vi "Append Waveform Data.vi"(8 "Count":i32, 10 "Data In":waveform(dbl), 11 "Data":waveform(dbl)) -> (3 "Data Out":waveform(dbl))   [LabVIEW 2018]
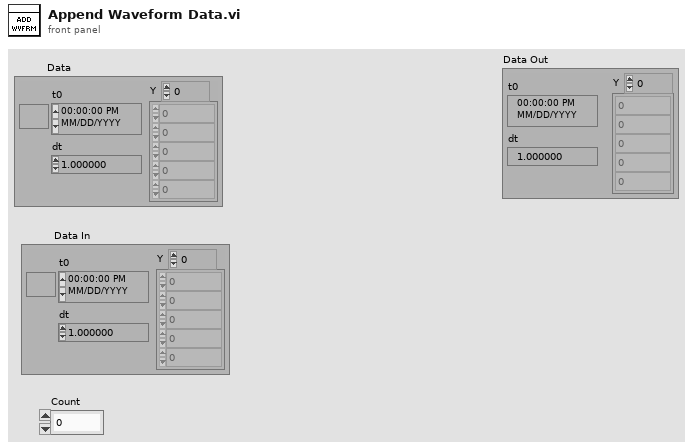
[diagram p1: front panel]
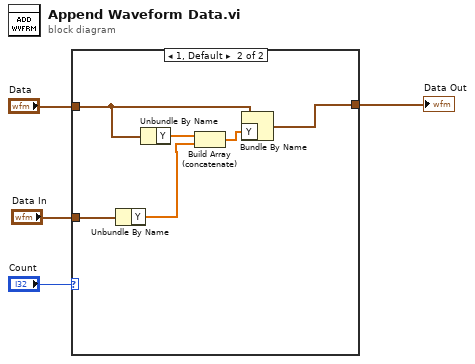
[diagram p0: block diagram]
diagram:
  n1 = case shown="1, Default" "Count" {
    tunnel: "Data" -> [_ w10]
    tunnel: [w5 w8] -> w3
    tunnel: "Data In" -> [w5 w7]
    frame 0 {
    }
    frame 1, Default {
      n2 = Unbundle By Name(w7) -> ("Y"=w6:dbl[])
      n3 = Unbundle By Name(w10) -> ("Y"=w11:dbl[])
      n4 = Build Array (concatenate)(w11, w6) -> (w9:dbl[])
      n5 = Bundle By Name(cluster=w10, "Y"=w9) -> (w8:waveform(dbl))
    }
  }
  "Data Out" <- w3
